vi "Mag_reading.vi"(8 "error in (no error)":errorcluster, 11 "VISA Mag in":refnum<visa-resource-name>) -> (0 "error out":errorcluster, 1 "Field magnitude (uT)":dbl, 3 "VISA Mag out":refnum<visa-resource-name>)   [LabVIEW 2017]
panel:
  out "after substring":string
  in  "Command 3":string="<?xml version=\"1.0\" encoding=\"ISO-8859-1\"?><cmd><instruction>GET_SAMPLE</instruction><md5>d8dd6be74a3df920ca20b397a0f49bc0</md5></cmd>"
  # "<?xml version=\"1.0\" encoding=\"ISO-8859-1\"?><reply><result><instruction>GET_SAMPLE</instruction><field_type>1</field_type><unit>8</unit><value>38.660324</value><x>4.975090</x><y>8.578482</y><z>37.366814</z><avg>38.424679</avg><peak>45.238209</peak><px>6.044888</px><py>8.796453</py><pz>43.961090</pz><f_cursor></f_cursor><sys_tick>81126038</sys_tick><gps_lat_deg></gps_lat_deg><gps_lon_deg></gps_lon_deg><gps_pdop></gps_pdop><gps_height></gps_height><probe_overrange>0</probe_overrange><probe_gain_changed>0</probe_gain_changed></result><md5>A383AE0CDC80D7E7DB1A0A1B39EF5EAD</md5></reply>"
  # "GET_SAMPLE:\n\n<?xml version=\"1.0\" encoding=\"ISO-8859-1\"?><cmd><instruction>GET_SAMPLE</instruction><md5>d8dd6be74a3df920ca20b397a0f49bc0</md5></cmd>"
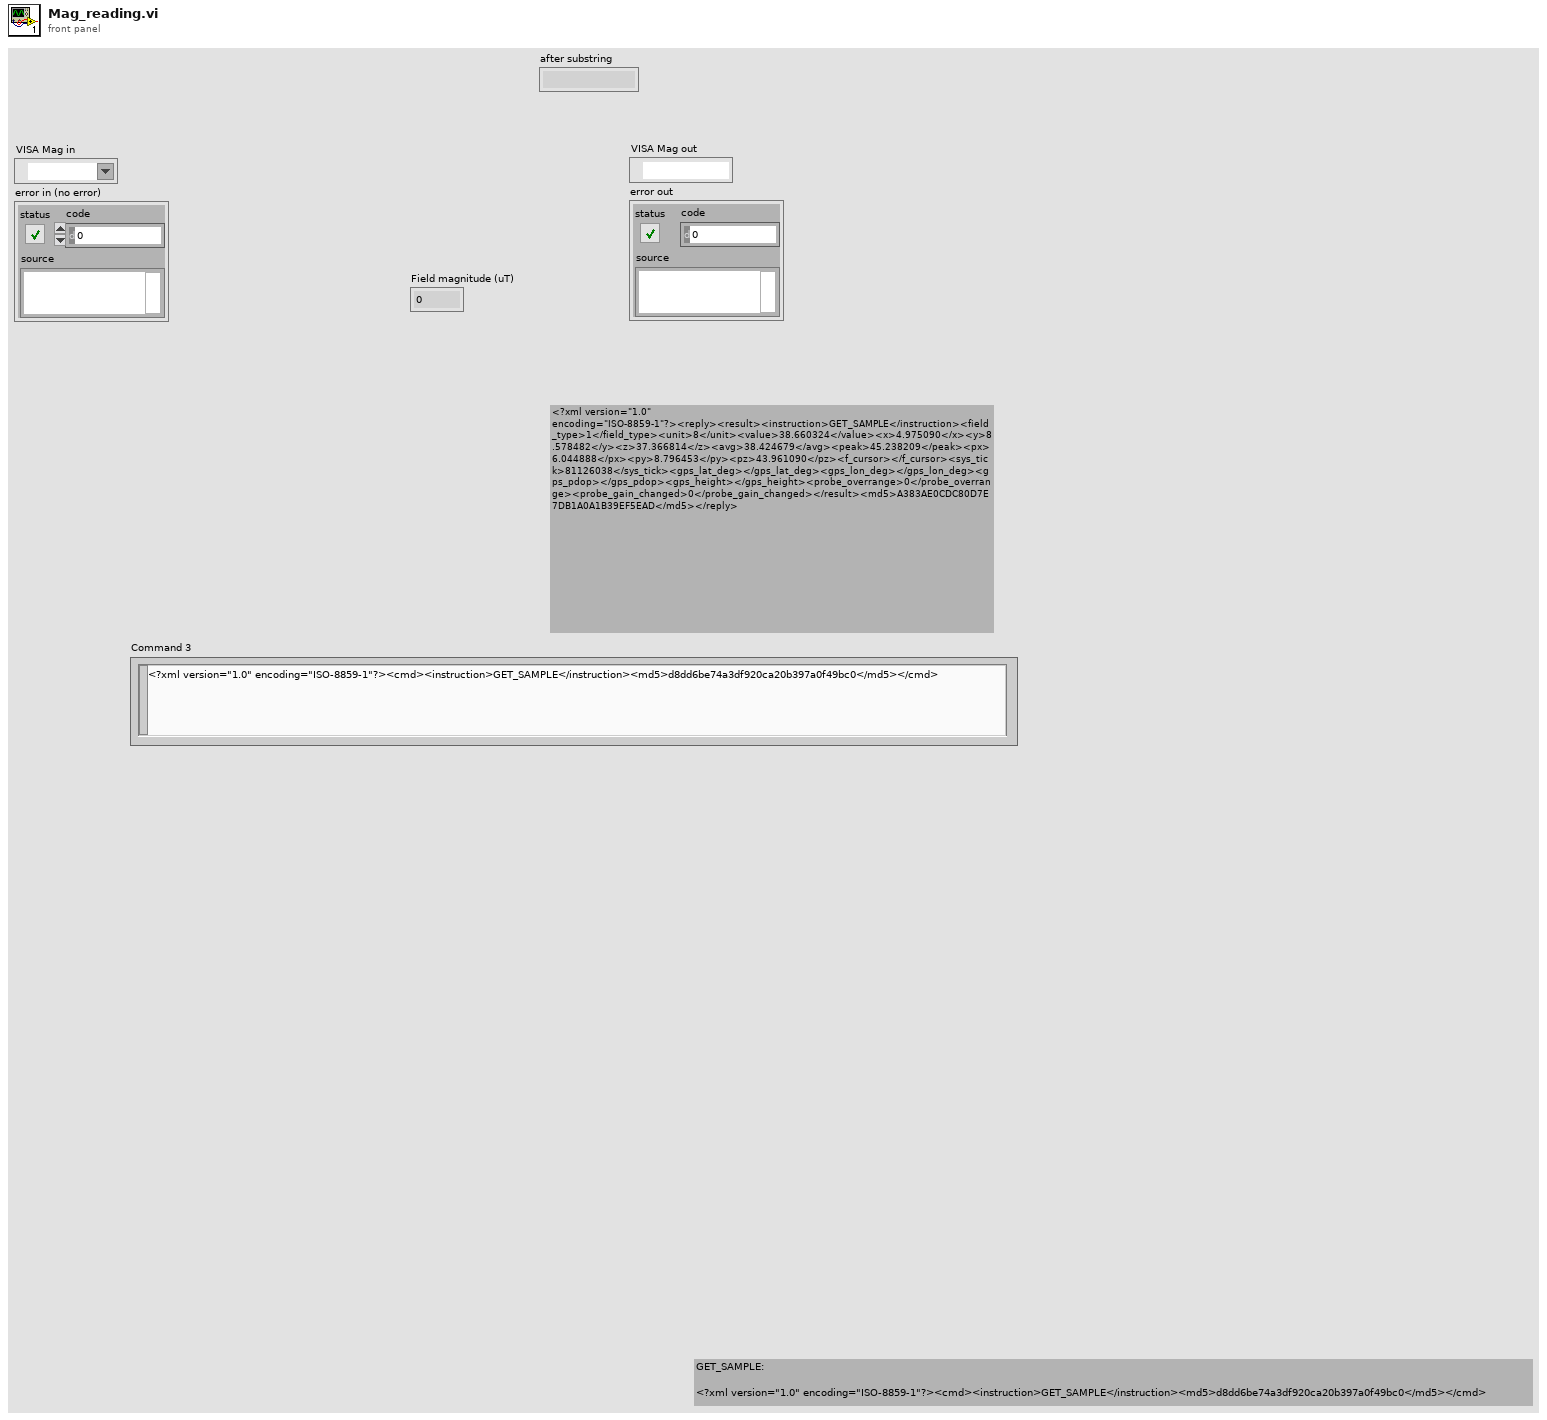
[diagram p1: front panel]
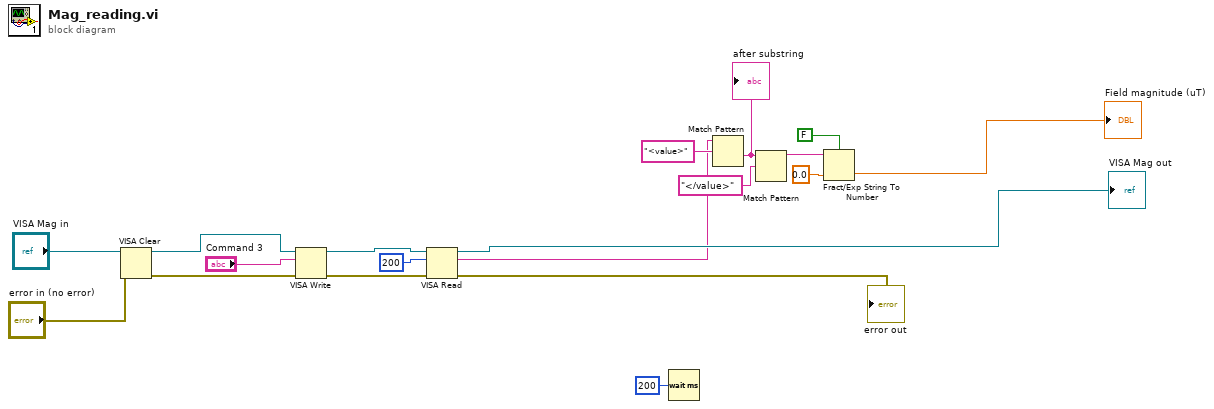
[diagram p0: block diagram]
diagram:
  n1 = VISA Clear(VISA resource name="VISA Mag in", error in (no error)="error in (no error)") -> (VISA resource name out=w17:refnum<visa-resource-name>, error out=w16:errorcluster)
  n2 = VISA Write(VISA resource name=w17, write buffer="Command 3", error in (no error)=w16) -> (VISA resource name out=w19:refnum<visa-resource-name>, error out=w18:errorcluster)  [unwired: 1 out]
  n3 = VISA Read(VISA resource name=w19, byte count=u32 200 ("Read Count 3"), error in (no error)=w18) -> (VISA resource name out=→"VISA Mag out":refnum<visa-resource-name>, read buffer=w8:string, error out=→"error out":errorcluster)  [unwired: 1 out]
  n4 = Wait (ms)(milliseconds to wait=u32 200) -> ()  [unwired: 1 out]
  n5 = Match Pattern(string=w8, regular expression="<value>") -> (after substring=w10:string)  [unwired: 1 in, 3 out]
  "after substring" <- w10
  n6 = Match Pattern(string=w10, regular expression="</value>") -> (before substring=w5:string)  [unwired: 1 in, 3 out]
  n7 = Fract/Exp String To Number(use system decimal point (T)=FALSE, string=w5, default (0 dbl)=0.0 ("default (0 DBL)")) -> (number=→"Field magnitude (uT)":dbl)  [unwired: 1 in, 1 out]
